vi "Meas_Fast_FID_Bkgnd.vi"(3 "Mode":T5, 5 "Traverse line In":T2 {"Carrier_2 Q (l/min)" format="%#.2f"; "Row Duration (mins)" format="%#.1f"; "Row No" min=0; "Trace Gas Concentration (%)" min=0.0 format="%#_4f"; "Carrier_1 Q (l/min)" format="%#.2f"; "Tunnel Speed" format="%#.2f"; "Start X" format="%#.2f"; "Start Y" format="%#.2f"; "Start Z" format="%#.2f"; "End X" format="%#.2f"; "End Y" format="%#.2f"; "End Z" format="%#.2f"; "Averaging time (min)" min=0.0 format="%#.2f"}) -> (0 "Error Message":string, 1 "Status":T1, 2 "Traverse line Out":T2 {"Carrier_2 Q (l/min)" format="%#.2f"; "Row Duration (mins)" format="%#.1f"; "Row No" min=0; "Trace Gas Concentration (%)" min=0.0 format="%#_4f"; "Carrier_1 Q (l/min)" format="%#.2f"; "Tunnel Speed" format="%#.2f"; "Start X" format="%#.2f"; "Start Y" format="%#.2f"; "Start Z" format="%#.2f"; "End X" format="%#.2f"; "End Y" format="%#.2f"; "End Z" format="%#.2f"; "Averaging time (min)" min=0.0 format="%#.2f"})   [LabVIEW 2015]
uses:
  Gen Trav/Traverse_cluster.ctl
  Gen Trav/Spacing.ctl
  Controls/Multi_run_mode.ctl
  Controls/User_Specific_mode.ctl
  Gen Trav/Multi_Run_Status.ctl
  File/Setup_Filetype.ctl
  Gen Trav/Trav_mode.ctl
  Controls/Home.ctl
  Controls/Setup.ctl
  Controls/Save_Data.ctl
  Globals/Trav_pos_global.vi
  Globals/Preference_global.vi
  Globals/Gas_management_global.vi
  Globals/Meas_global.vi
panel:
  out "Traverses":string[](array[string])
  out "Initial Trav Positions":sgl[][](array[numeric])
  out "First Bknd since calib":bool
  out "Initial Position":sgl[](array[numeric]) format="%#.2f"
  # "X           Y            Z"
  # "Start"
  # "End"
  # "X           Y            Z"
  # "Start"
  # "End"
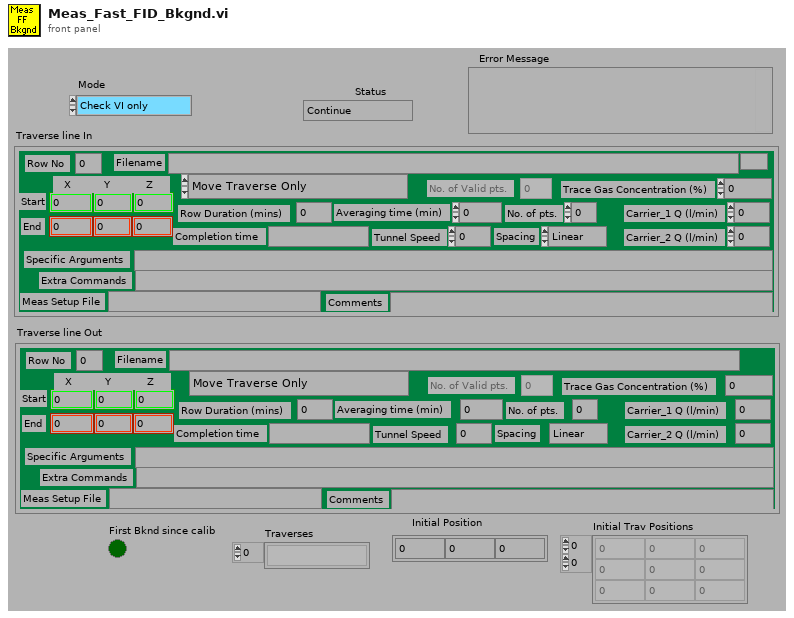
[diagram p1: front panel]
types:
  T1 = typedef "Multi_Run_Status.ctl" = enum16{"Continue", "Jump to Next Point", "Jump to Next Row", "Jump To Fall Back", "Terminate Run"}
  T2 = typedef "Traverse_cluster.ctl" = cluster{"Start X":sgl, "Start Y":sgl, "Start Z":sgl, "End X":sgl, "End Y":sgl, "End Z":sgl, "No. of pts.":i32, "Spacing":T3, "Filename":path, "Tunnel Speed":dbl, "Averaging time (min)":dbl, "Extra Commands":string, "Carrier_1 Q (l/min)":dbl, "Carrier_2 Q (l/min)":dbl, "Trace Gas Concentration (%)":dbl, "Specific Arguments":string, "Comments":string, "Row No":i32, "Row Type Selector":T4, "Completion time":string, "Row Duration (mins)":dbl, "No. of Valid pts.":i32, "Meas Setup File":string}
  T3 = typedef "Spacing.ctl" = enum16{"Linear", "Log", "Gauss", "Specified", "N/A"}
  T4 = typedef "Multi_run_mode.ctl" = enum16{"Move Traverse Only", "Set Tunnel Speed Only", "Set Source Only", "Set Measurement Conditions", "Single Measurement", "Vertical Profile", "Lateral Profile", "Longitudinal Profile", "Explore Volume", "Multi-Axis Profile", "Auto Calibrate", "Meas Fast FID Bkgnd", "Check Beam Power", "Scanning Valve Measurement", "Run VI Named:", "Set ADAM Ch", "Wait (minutes)", "Send Message", "Synchronize With:", "Fall Back to this Row", "Turn Off Row Repeating", "Blank Row", "Traverse 3D Volume"}
  T5 = typedef "User_Specific_mode.ctl" = enum16{"Check VI only", "Run VI"}
  T6 = typedef "Tunnel_Coordinates.ctl" = enum16{"Work in Tunnel Coordinates", "Work in Model Coordinates"}
  T7 = typedef "Setup_Filetype.ctl" = enum16{"Measurement Setups", "Calibration Setups", "General", "Results File Plotter Setups", "Speed Calib Tweaks"}
  T8 = typedef "Trav_mode.ctl" = enum16{"Move traverse", "Read traverse position", "Teach Position"}
  T9 = typedef "Home.ctl" = enum16{"Don't Home", "Home  +X", "Home  -X", "Home  +Y", "Home  -Y", "Home  +Z", "Home  -Z"}
  T10 = typedef "Save_Data.ctl" = enum16{"Save No Data", "Save Data"}
  T11 = typedef "Setup.ctl" = enum16{"Run Program", "Show Setup", "Save Current Setup", "Setup Front Panel"}
  T12 = typedef "Status_Cluster.ctl" = cluster{"Status":T1, "Error Type":string, "Error Description":string}
  T13 = typedef "Analysis_info_cluster.ctl" = cluster{"Colour":u32, "Inst type":T14, "Inst name":string, "Symbol":string, "Code name":string, "Extra Info":string, "Inst Array":T15, "Extra Titles":string[], "Extra Values":string[], "U":dbl, "u^2":dbl, "u^3":dbl, "u^4":dbl, "Skew_u":dbl, "Kurt_u":dbl, "Sd Error in Mean":dbl, "% u'/U":dbl, "X":dbl, "Y":dbl, "Z":dbl, "Timescale integral to 25%":dbl, "Sd Error in Variance":dbl, "Calib File":path, "Calib Constants":dbl[], "Output Position":bool, "Full Stats":bool, "Av Sampling Rate":dbl, "Av No of Samples":dbl, "Total Meas Time (s)":dbl, "ADAM Ch Name":string, "Max value":dbl, "Min value":dbl}
  T14 = typedef "Inst_type.ctl" = enum16{"Propeller anemometer", "Raw voltage", "Pressure Transducer", "Pitot-static tube", "Preston tube", "Hot wire", "Cross wire 1", "Cross wire 2", "Generic Linear", "Generic Polynomial", "Generic BackPoly", "Fast FID", "Thermocouple", "Cold wire", "Pulsed Wire", "LDA Vel", "LDA Tran time", "LDA Arr time", "Microphone"}
  T15 = typedef "Instrument_Array.ctl" = enum16{"PWA", "LDA", "Analogue"}
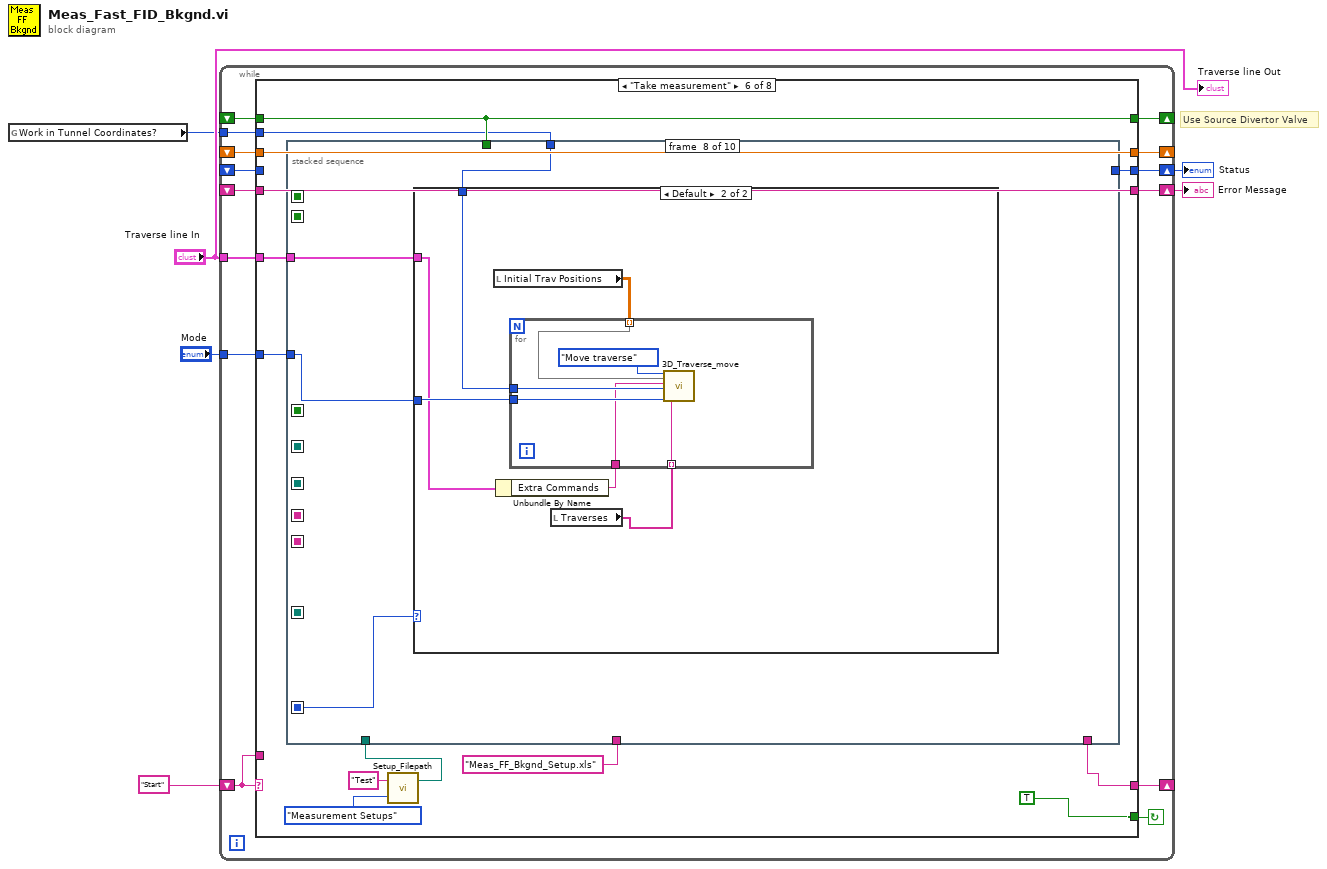
[diagram p0: block diagram]
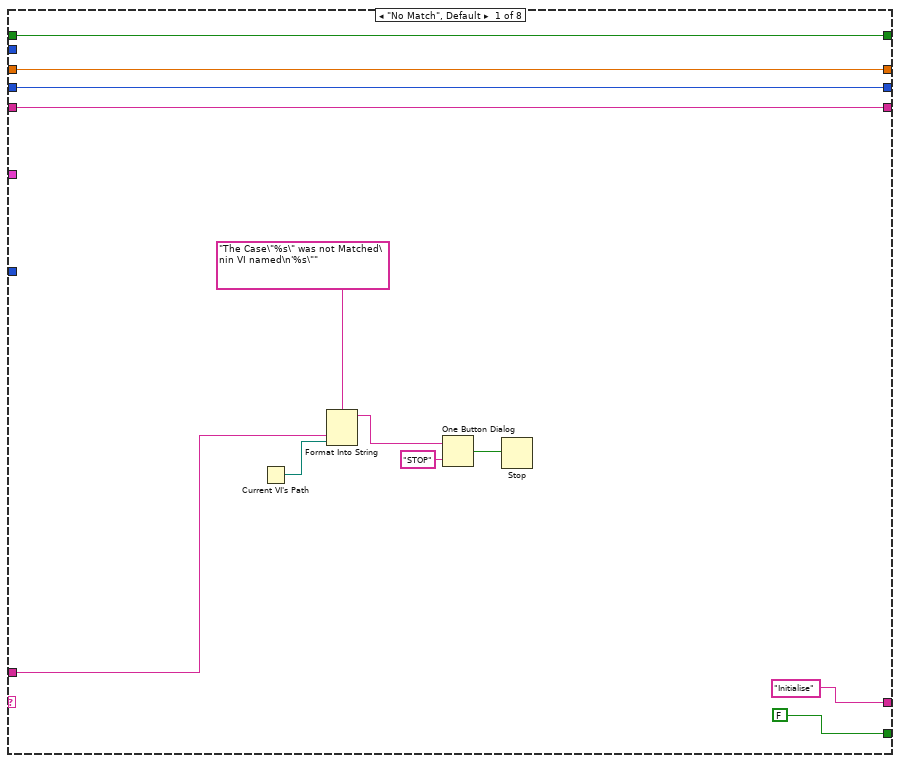
[diagram p2: hidden frame]
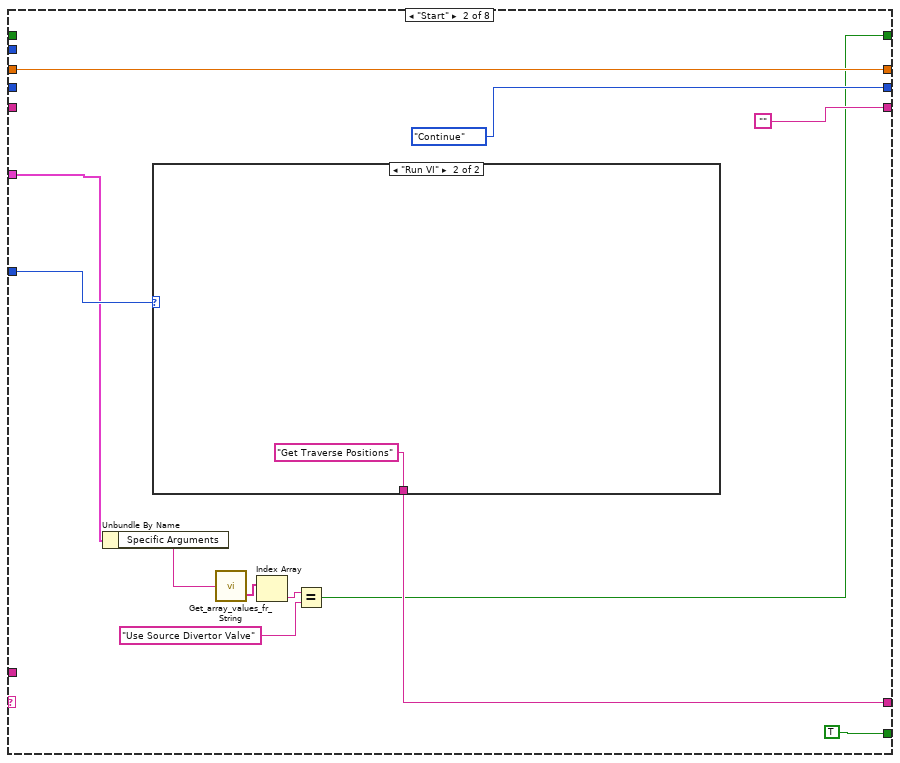
[diagram p3: hidden frame]
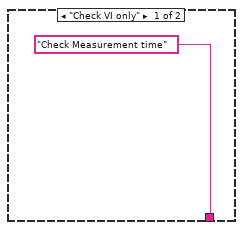
[diagram p4: hidden frame]
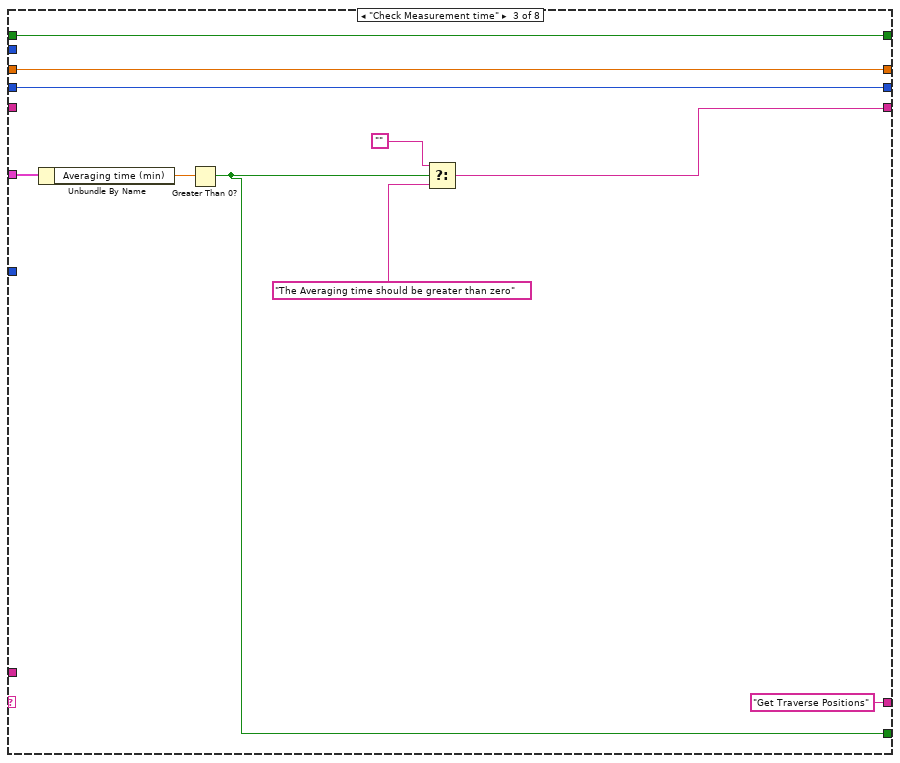
[diagram p5: hidden frame]
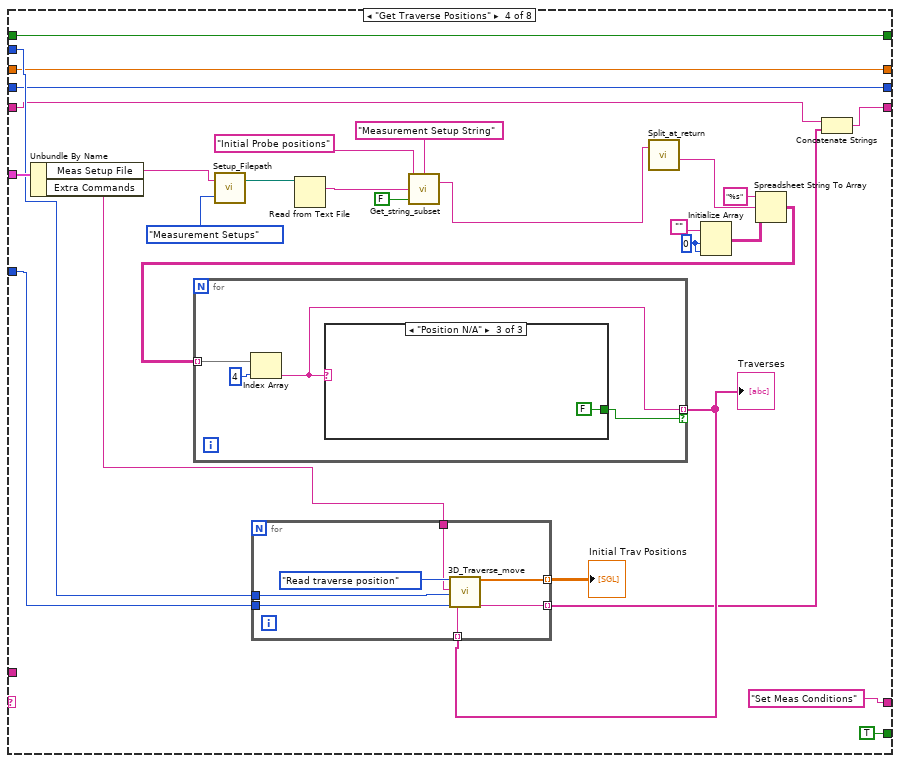
[diagram p6: hidden frame]
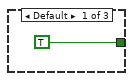
[diagram p7: hidden frame]
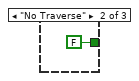
[diagram p8: hidden frame]
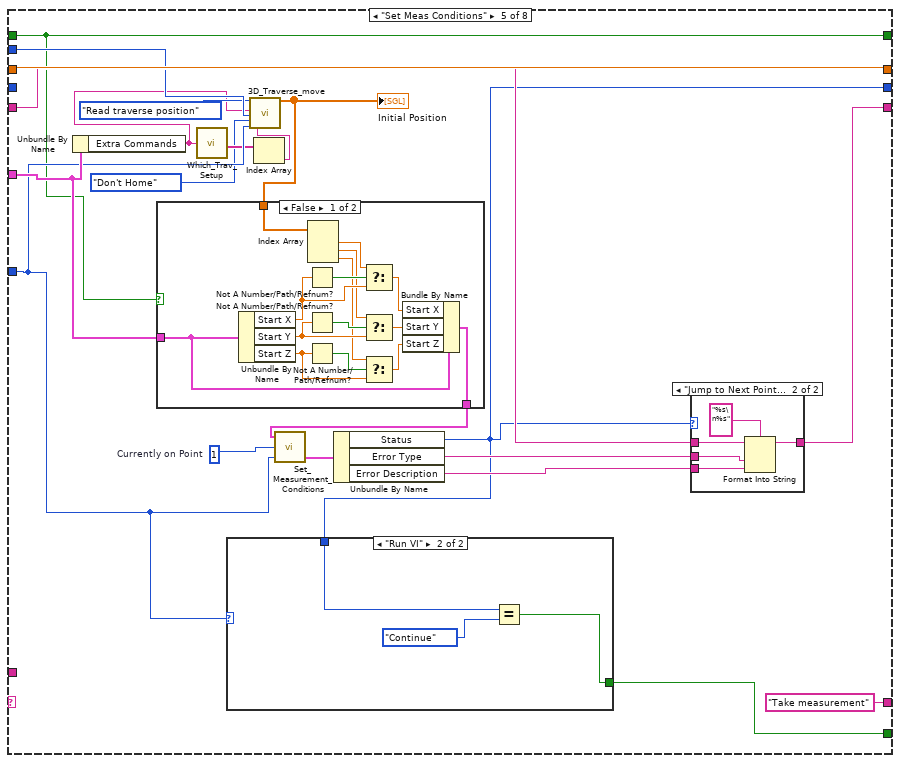
[diagram p9: hidden frame]
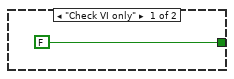
[diagram p12: hidden frame]
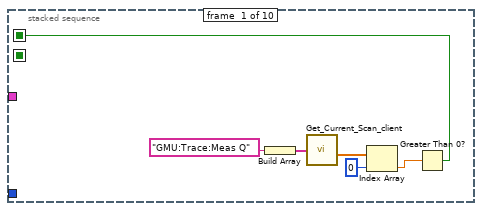
[diagram p13: hidden frame]
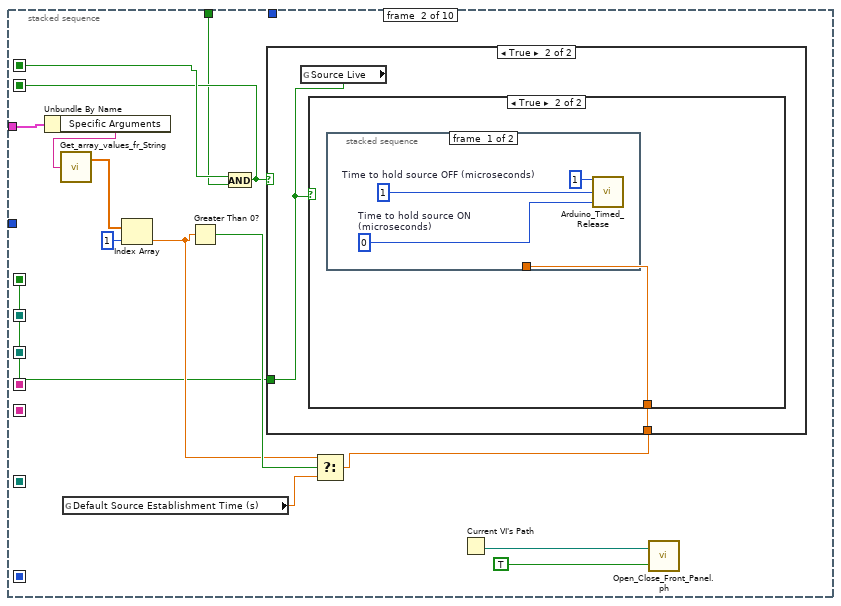
[diagram p14: hidden frame]
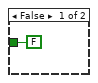
[diagram p15: hidden frame]
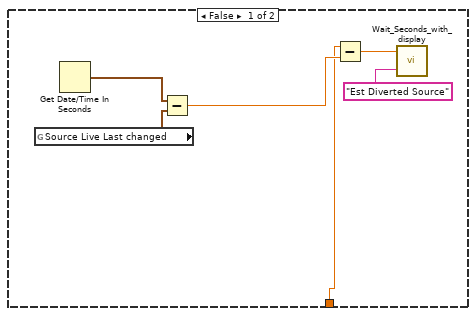
[diagram p16: hidden frame]
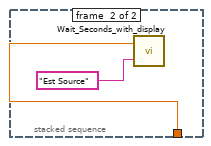
[diagram p17: hidden frame]
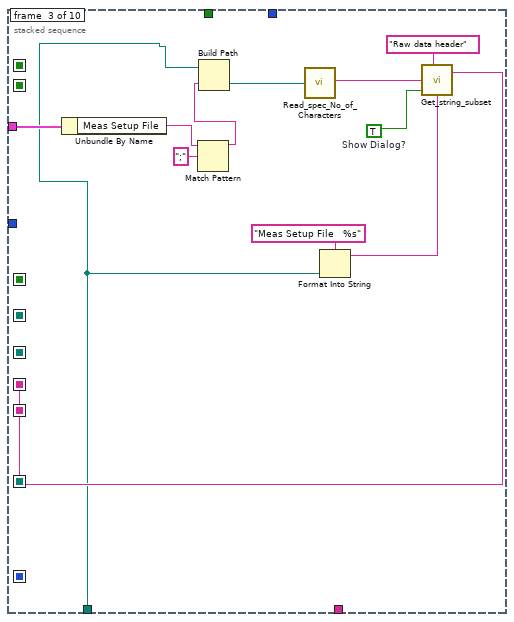
[diagram p18: hidden frame]
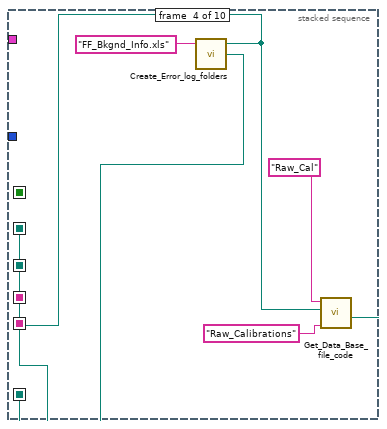
[diagram p19: hidden frame]
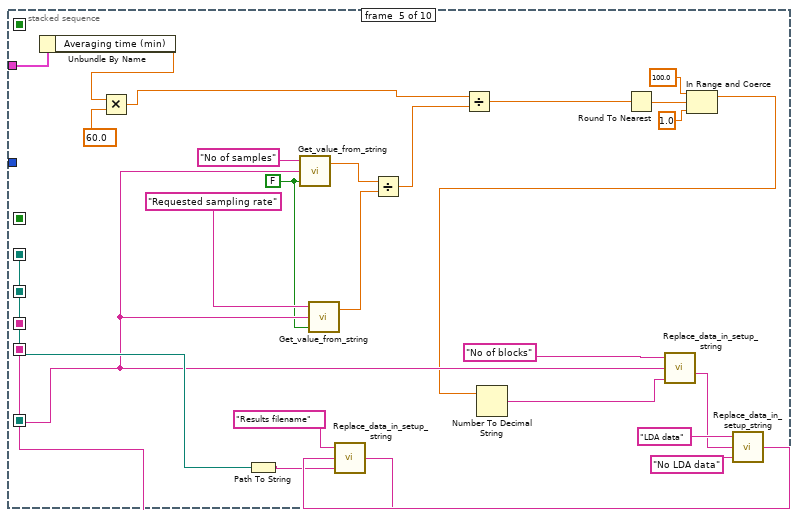
[diagram p20: hidden frame]
diagram:
  # "Use Source Divertor Valve"
  n1 = global read "Trav_pos_global.vi" "Work in Tunnel Coordinates?"() -> (w1:T6)
  n2 = while {
    shift-left: "Start" -> [w18]
    shift-right: [w19] -> _
    shift-right: [w14] -> _
    shift-left: _ -> [w17]
    tunnel: "Mode" -> [w16]
    tunnel: "Traverse line In" -> [w15]
    shift-right: [w13] -> w4
    shift-left: _ -> [w11]
    shift-right: [w12] -> w2
    shift-left: _ -> [w10]
    tunnel: w1 -> [w9]
    shift-right: [w7] -> _
    shift-left: _ -> [w8]
    stop <- w20 continue-if-true
    n3 = case shown="\"Take measurement\"" w18 {
      tunnel: [FALSE TRUE w50 TRUE w112 TRUE TRUE FALSE] -> w20
      tunnel: ["Initialise" w42 "Get Traverse Positions" "Set Meas Conditions" "Take measurement" ("t") w152 "Reset Measurement Program" "End"] -> w19
      tunnel: w18 -> [w27 _ _ _ _ _ _ _]
      tunnel: w17 -> [w24 w40 w48 w63 w117 w157 w393 _]
      tunnel: w16 -> [_ w43 _ w65 w108 w147 _ _]
      tunnel: w15 -> [_ w36 w56 w83 w109 w155 _ _]
      tunnel: [w24 w40 w48 w63 w117 w157 w393 w398] -> w14
      tunnel: [w23 Multi_Run_Status."Continue" ("Status") w49 w62 w110 w153 w392 w397] -> w13
      tunnel: [w22 "" w52 w59 w113 w156 w391 w400] -> w12
      tunnel: w11 -> [w23 _ w49 w62 _ _ w392 w397]
      tunnel: w10 -> [w22 _ _ w61 w114 w156 w391 w400]
      tunnel: w9 -> [_ _ _ w64 w107 w146 _ _]
      tunnel: w8 -> [w21 _ w47 w84 w99 w148 w388 w396]
      tunnel: [w21 w34 w47 w84 w99 w148 w388 w396] -> w7
      frame "No Match", Default {
        n4 = Current VI's Path() -> (path=w26:path)
        n5 = Format Into String(format string="The Case\"%s\" was not Matched\nin VI named\n'%s\"" ("Format String"), w27, w26) -> (resulting string=w30:string)  [unwired: 2 in, 1 out]
        n6 = One Button Dialog(message=w30, button name ("OK")="STOP") -> (true=w28:bool)
        n7 = Stop(stop? (T)=w28) -> ()
      }
      frame "Start" {
        n8 = Unbundle By Name(w36) -> ("Specific Arguments"=w35:string)
        n9 = case shown="\"Run VI\"" w43 {
          tunnel: ["Check Measurement time" "Get Traverse Positions"] -> w42
          frame "Check VI only" {
          }
          frame "Run VI" {
          }
        }
        n10 = call "Get_array_values_fr_String.vi"("String Value"=w35) -> ("String array"=w38:string[])  [unwired: 1 out]
        n11 = Index Array(array=w38) -> (element=w37:string)  [unwired: 1 in]
        n12 = Equal?(x=w37, y="Use Source Divertor Valve") -> (x = y?=w34:bool)
      }
      frame "Check Measurement time" {
        n13 = Unbundle By Name(w56) -> ("Averaging time (min)"=w55:dbl)
        n14 = Greater Than 0?(x=w55) -> (x > 0?=w50:bool)
        n15 = Select(t="", s=w50, f="The Averaging time should be greater than zero") -> (s? t:f=w52:string)
      }
      frame "Get Traverse Positions" {
        w77 = 0 ("Dimension Size")
        n16 = Unbundle By Name(w83) -> ("Meas Setup File"=w81:string, "Extra Commands"=w66:string)
        n17 = call "Setup_Filepath.vi"("Setup File Type"=Setup_Filetype."Measurement Setups", "Filename in"=w81) -> ("Directory"=w80:path)  [unwired: 1 out]
        n18 = Read from Text File(file (use dialog)=w80) -> (text=w70:string)  [unwired: 3 in, 3 out]
        n19 = call "Get_string_subset.vi"("String Name"="Measurement Setup String", "Show Dialog?"=FALSE, "String to split"=w70, "File Label"="Initial Probe positions") -> ("Output string"=w79:string)  [unwired: 1 out]
        n20 = call "Split_at_return.vi"("String"=w79) -> ("after substring"=w74:string)  [unwired: 1 in, 3 out]
        n21 = Initialize Array("", w77, w77) -> (w78:string[][])
        n22 = Spreadsheet String To Array(format string="%s", spreadsheet string=w74, array type (2D Dbl)=w78) -> (array=w69:string[][])  [unwired: 1 out]
        n23 = for {
          tunnel: w69 -> [w94] mode=indexing
          tunnel: [w93] -> w67 mode=indexing if=w92
          n24 = Index Array(array=w94, index=4) -> (element=w93:string)
          n25 = case shown="\"Position N/A\"" w93 {
            tunnel: [TRUE FALSE FALSE] -> w92
            frame Default {
            }
            frame "No Traverse" {
            }
            frame "Position N/A" {
            }
          }
        }
        "Traverses" <- w67
        n26 = for {
          tunnel: w67 -> [w90] mode=indexing
          tunnel: w64 -> [w89]
          tunnel: w66 -> [w88]
          tunnel: w65 -> [w87]
          tunnel: [w86] -> w68 mode=indexing
          tunnel: [w85] -> w60 mode=indexing
          n27 = call "3D_Traverse_move.vi"("Mode"=Trav_mode."Read traverse position", "Extra command String"=w88, "Work in Tunnel Coordinates"=w89, "Simulate/Run"=w87, "Traverse name"=w90) -> ("Trav Position achieved"=w86:sgl[], "Error String"=w85:string)  [unwired: 12 in, 1 out]
        }
        "Initial Trav Positions" <- w68
        n28 = Concatenate Strings(w61, w60) -> (w59:string)
      }
      frame "Set Meas Conditions" {
        w119 = 1  # Currently on Point
        n29 = Unbundle By Name(w109) -> ("Extra Commands"=w100:string)
        n30 = call "Which_Trav_Setup.vi"("Extra Command String"=w100) -> ("Traverse Setups"=w103:string[])
        n31 = Index Array(array=w103) -> (element=w102:string)  [unwired: 1 in]
        n32 = call "3D_Traverse_move.vi"("Mode"=Trav_mode."Read traverse position", "Extra command String"=w100, "Work in Tunnel Coordinates"=w107, "Home"=Home."Don't Home", "Simulate/Run"=w108, "Traverse name"=w102) -> ("Trav Position achieved"=w104:sgl[])  [unwired: 11 in, 2 out]
        "Initial Position" <- w104
        n33 = case shown="False" w99 {
          tunnel: w109 -> [w134 w135]
          tunnel: [w133 w135] -> w106
          tunnel: w104 -> [w132 _]
          frame False {
            n34 = Unbundle By Name(w134) -> ("Start X"=w128:sgl, "Start Y"=w124:sgl, "Start Z"=w123:sgl)
            n35 = Not A Number/Path/Refnum?(number/path/refnum=w128) -> (NaN/Path/Refnum?=w131:bool)
            n36 = Not A Number/Path/Refnum?(number/path/refnum=w124) -> (NaN/Path/Refnum?=w127:bool)
            n37 = Not A Number/Path/Refnum?(number/path/refnum=w123) -> (NaN/Path/Refnum?=w126:bool)
            n38 = Index Array(array=w132) -> (element #1=w129:sgl, element #2=w122:sgl, element #3=w121:sgl)  [unwired: 3 in]
            n39 = Select(t=w129, s=w131, f=w128) -> (s? t:f=w130:sgl)
            n40 = Select(t=w122, s=w127, f=w124) -> (s? t:f=w125:sgl)
            n41 = Select(t=w121, s=w126, f=w123) -> (s? t:f=w120:sgl)
            n42 = Bundle By Name(cluster=w134, "Start X"=w130, "Start Y"=w125, "Start Z"=w120) -> (w133:T2)
          }
          frame True {
          }
        }
        n43 = call "Set_Measurement_Conditions.vi"("Simulate/Run"=w108, "Currently on Point"=w119, "Traverse line"=w106) -> ("Status Cluster"=w118:T12)  [unwired: 2 out]
        n44 = Unbundle By Name(w118) -> ("Status"=w110:T1, "Error Type"=w116:string, "Error Description"=w115:string)
        n45 = case shown="\"Run VI\"" w108 {
          tunnel: [FALSE w144] -> w112
          tunnel: w110 -> [_ w145]
          frame "Check VI only" {
          }
          frame "Run VI" {
            n46 = Equal?(x=w145, y=Multi_Run_Status."Continue" ("Status")) -> (x = y?=w144:bool)
          }
        }
        n47 = case shown="\"Jump to Next Point\", Default" w110 {
          tunnel: w116 -> [_ w141]
          tunnel: w115 -> [_ w140]
          tunnel: w114 -> [w136 w139]
          tunnel: [w136 w138] -> w113
          frame "Continue" {
          }
          frame "Jump to Next Point", Default {
            n48 = Format Into String(format string="%s\n%s", initial string=w139, w141, w140) -> (resulting string=w138:string)  [unwired: 1 in, 1 out]
          }
        }
      }
      frame "Take measurement" {
        n49 = call "Setup_Filepath.vi"("Setup File Type"=Setup_Filetype."Measurement Setups", "Filename in"="Test") -> ("Directory"=w149:path)  [unwired: 1 out]
        n50 = stacked-sequence {
          seq-local: [_ _ w203 _ _ _ _ _ _ _] -> [_ _ _ _ w219 _ _ _ _ _]
          seq-local: [_ _ _ _ w228 _ _ _ _ _] -> [_ _ _ _ _ w240 _ _ _ _]
          seq-local: [_ _ _ w208 _ _ _ _ _ _] -> [_ _ _ _ _ _ w259 _ _ _]
          seq-local: [_ _ _ w210 _ _ _ _ _ _] -> [_ _ _ _ w227 _ _ _ w372 _]
          seq-local: [_ w167 _ _ _ _ _ _ _ _] -> [_ _ _ _ _ _ _ _ _ _]
          seq-local: [_ _ _ w207 _ _ _ _ _ _] -> [_ _ _ _ _ _ _ _ w371 _]
          seq-local: [w159 _ _ _ _ _ _ _ _ _] -> [_ w168 _ _ _ _ _ _ _ _]
          seq-local: [_ w165 _ _ _ _ _ _ _ _] -> [_ _ _ _ _ _ _ _ w370 _]
          seq-local: [_ _ _ _ _ _ w249 _ _ _] -> [_ _ _ _ _ _ _ w357 _ _]
          tunnel: "Meas_FF_Bkgnd_Setup.xls" -> [_ _ _ _ _ w242 w260 _ _ _]
          tunnel: w155 -> [_ w176 w200 _ w223 _ w252 w356 _ w378]
          tunnel: [_ _ _ _ _ _ w258 _ _ _] -> w153
          tunnel: [_ _ _ _ _ _ w256 _ _ _] -> w152
          tunnel: w149 -> [_ _ w195 _ _ w238 _ _ _ _]
          tunnel: w148 -> [_ w166 _ _ _ _ _ _ _ _]
          tunnel: w147 -> [_ _ _ _ _ _ w250 w355 _ w377]
          tunnel: w146 -> [_ _ _ _ _ _ w251 w354 _ _]
          frame #0 {
            n51 = Build Array("GMU:Trace:Meas Q") -> (w163:string[])
            n52 = call "Get_Current_Scan_client.vi"("ADAM Ch Names"=w163) -> ("Numerical Values"=w161:dbl[])  [unwired: 3 out]
            n53 = Index Array(array=w161, index=0) -> (element=w160:dbl)
            n54 = Greater Than 0?(x=w160) -> (x > 0?=w159:bool)
          }
          frame #1 {
            n55 = Unbundle By Name(w176) -> ("Specific Arguments"=w175:string)
            n56 = call "Get_array_values_fr_String.vi"("String Value"=w175) -> ("Numeric Array"=w173:dbl[])  [unwired: 1 out]
            n57 = global read "Preference_global.vi" "Default Source Establishment Time (s)"() -> (w170:dbl)
            n58 = Index Array(array=w173, index=1) -> (element=w171:dbl)
            n59 = Greater Than 0?(x=w171) -> (x > 0?=w172:bool)
            n60 = And(x=w168, y=w166) -> (x .and. y?=w167:bool)
            n61 = Select(t=w171, s=w172, f=w170) -> (s? t:f=w169:dbl)
            n62 = case shown="True" w167 {
              tunnel: w169 -> [_ w181]
              tunnel: [FALSE w180] -> w165
              frame False {
              }
              frame True {
                n63 = global read "Gas_management_global.vi" "Source Live"() -> (w180:bool)
                n64 = case shown="True" w180 {
                  tunnel: w181 -> [w182 w188]
                  frame False {
                    n65 = global read "Gas_management_global.vi" "Source Live Last changed"() -> (w184:timestamp)
                    n66 = Get Date/Time In Seconds() -> (seconds since 1Jan1904=w183:timestamp)
                    n67 = Subtract(x=w183, y=w184) -> (x-y=w185:dbl)
                    n68 = Subtract(x=w182, y=w185) -> (x-y=w187:dbl)
                    n69 = call "Wait_Seconds_with_display.vi"("Message"="Est Diverted Source", "Seconds to wait"=w187) -> ()  [unwired: 2 out]
                  }
                  frame True {
                    n70 = stacked-sequence {
                      tunnel: w188 -> [_ w192]
                      frame #0 {
                        w189 = u32 1  # Time to hold source OFF (microseconds)
                        w190 = u32 0  # Time to hold source ON (microseconds)
                        n71 = call "Arduino_Timed_Release.vi"("Time to hold source ON (microseconds)"=w190, "Time to hold source OFF (microseconds)"=w189, "Number of cycles"=u16 1) -> ()  [unwired: 2 out]
                      }
                      frame #1 {
                        n72 = call "Wait_Seconds_with_display.vi"("Message"="Est Source", "Seconds to wait"=w192) -> ()  [unwired: 2 out]
                      }
                    }
                  }
                }
              }
            }
            n73 = Current VI's Path() -> (path=w177:path)
            n74 = call "Open_Close_Front_Panel.ph.vi"("Front Panel Window:Open"=TRUE, "VI path"=w177) -> ()  [unwired: 2 out]
          }
          frame #2 {
            w201 = TRUE  # Show Dialog?
            n75 = Unbundle By Name(w200) -> ("Meas Setup File"=w198:string)
            n76 = Match Pattern(string=w198, regular expression=";") -> (before substring=w197:string)  [unwired: 4 out]
            n77 = Build Path(base path=w195, name or relative path=w197) -> (appended path=w202:path)
            n78 = call "Read_spec_No_of_Characters.vi"("Filename"=w202) -> ("character string"=w204:string)  [unwired: 1 out]
            n79 = Format Into String(format string="Meas Setup File   %s", w195) -> (resulting string=w194:string)  [unwired: 2 in, 1 out]
            n80 = call "Get_string_subset.vi"("String Name"=w194, "Show Dialog?"=w201, "String to split"=w204, "File Label"="Raw data header") -> ("Output string"=w203:string)  [unwired: 1 out]
          }
          frame #3 {
            n81 = call "Create_Error_log_folders.vi"("Log Filename"="FF_Bkgnd_Info.xls") -> ("Server copy Location"=w207:path, "Local Log File"=w210:path)  [unwired: 2 in, 1 out]
            n82 = call "Get_Data_Base_file_code.vi"("Data Type"="Raw_Calibrations", "Results Filename"=w210, "Short_Name"="Raw_Cal") -> ("Raw Data File Name"=w208:path)  [unwired: 1 in, 3 out]
          }
          frame #4 {
            w216 = FALSE ("Show Dialog?")
            n83 = Unbundle By Name(w223) -> ("Averaging time (min)"=w222:dbl)
            n84 = Multiply(x=w222, y=60.0) -> (x*y=w224:dbl)
            n85 = Path To String(path=w227) -> (string=w226:string)
            n86 = call "Get_value_from_string.vi"("Show Dialog?"=w216, "Input string"=w219, "Variable name"="No of samples") -> ("Value"=w217:dbl)  [unwired: 1 out]
            n87 = call "Get_value_from_string.vi"("Show Dialog?"=w216, "Input string"=w219, "Variable name"="Requested sampling rate") -> ("Value"=w218:dbl)  [unwired: 1 out]
            n88 = Divide(x=w217, y=w218) -> (x/y=w237:dbl)
            n89 = Divide(x=w224, y=w237) -> (x/y=w236:dbl)
            n90 = Round To Nearest(number=w236) -> (nearest integer value=w215:dbl)
            n91 = In Range and Coerce(upper limit=100.0, x=w215, lower limit=1.0) -> (coerced(x)=w212:dbl)  [unwired: 1 out]
            n92 = Number To Decimal String(number=w212) -> (decimal integer string=w234:string)  [unwired: 1 out]
            n93 = call "Replace_data_in_setup_string.vi"("New data string"=w234, "Input string"=w219, "Variable name"="No of blocks") -> ("Appended string"=w231:string)
            n94 = call "Replace_data_in_setup_string.vi"("New data string"="No LDA data", "Input string"=w231, "Variable name"="LDA data" ("Label for characters")) -> ("Appended string"=w229:string)
            n95 = call "Replace_data_in_setup_string.vi"("New data string"=w226, "Input string"=w229, "Variable name"="Results filename") -> ("Appended string"=w228:string)
          }
          frame #5 {
            w246 = FALSE  # advisory dialog? (display:T)
            w247 = FALSE  # append to file? (new file:F)
            n96 = call "Remove_Plug_Ins_etc.vi"("Input String"=w240) -> ("Output string"=w239:string)
            n97 = call "Add_label_to_string.vi"("String to write"=w239, "File Label"="Raw data header") -> ("Output string"=w243:string)
            n98 = Build Path(base path=w238, name or relative path=w242) -> (appended path=w241:path)
            n99 = call "Add_length_to_string.vi"("String in"=w243) -> ("String out"=w245:string)
            n100 = call "Write_Characters_To_File.vi"("file path (dialog if empty)"=w241, "advisory dialog? (display:T)"=w246, "character string"=w245, "append to file? (new file:F)"=w247) -> ()  [unwired: 1 in, 4 out]
          }
          frame #6 {
            n101 = for {
              N: 4 -> [_]
              tunnel: w260 -> [w270]
              tunnel: w259 -> [w269]
              tunnel: [w268] -> w258
              tunnel: [w267] -> w257
              tunnel: w252 -> [w265]
              tunnel: w251 -> [w264]
              tunnel: w250 -> [w263]
              tunnel: [w262] -> w249
              tunnel: [w261] -> w248
              i -> [w262]
              stop <- w266 continue-if-true
              n102 = stacked-sequence {
                seq-local: [w273 _ _ _ _] -> [_ _ w308 _ _]
                seq-local: [_ _ w307 _ _] -> [_ _ _ w313 w331]
                seq-local: [_ w284 _ _ _] -> [_ _ w306 _ _]
                tunnel: w270 -> [w279 _ _ _ _]
                tunnel: w269 -> [w277 _ _ _ _]
                tunnel: [w275 _ _ _ _] -> w268
                tunnel: [w273 _ _ _ _] -> w267
                tunnel: [_ _ w307 _ _] -> w266
                tunnel: w265 -> [w271 _ _ w312 w330]
                tunnel: w264 -> [_ _ _ w311 w329]
                tunnel: w263 -> [_ _ _ w310 w328]
                tunnel: w262 -> [_ _ _ w309 w327]
                tunnel: [_ w282 _ _ _] -> w261
                frame #0 {
                  w281 = TRUE  # Remote control
                  n103 = Unbundle By Name(w271) -> ("Extra Commands"=w272:string)
                  n104 = call "Code_to_run.vi"("Extra command String"=w272, "Raw data option"=enum16{"Save raw data", "Raw data not saved"}."Save raw data", "setup"=Setup."Run Program", "Remote control"=w281, "File"=Save_Data."Save Data", "Raw data file"=w277, "Setup filename"=w279) -> ("Status"=w275:T1)  [unwired: 5 in, 3 out]
                  n105 = Equal?(x=w275, y=Multi_Run_Status."Continue" ("Status")) -> (x = y?=w273:bool)
                }
                frame #1 {
                  n106 = global read "Meas_global.vi" "Analysis Info cluster"() -> (w286:T13[])
                  n107 = for {
                    tunnel: w286 -> [w289] mode=indexing
                    tunnel: [w288] -> w285 mode=indexing
                    tunnel: [w287] -> w283 mode=indexing
                    n108 = Unbundle By Name(w289) -> ("Inst type"=w290:T14)
                    n109 = case shown="\"Fast FID\"" w290 {
                      tunnel: w289 -> [_ w305]
                      tunnel: [FALSE w294] -> w288
                      tunnel: [FALSE w293] -> w287
                      frame Default {
                      }
                      frame "Fast FID" {
                        n110 = Unbundle By Name(w305) -> ("u^2"=w300:dbl, "Calib Constants"=w301:dbl[])
                        n111 = Index Array(array=w301, index=3 ("Index")) -> (element=w303:dbl)
                        n112 = Index Array(array=w301, index=4) -> (element=w297:dbl)
                        n113 = Equal To 0?(x=w303) -> (x = 0?=w293:bool)
                        n114 = Multiply(x=w297, y=1.4) -> (x*y=w295:dbl)
                        n115 = Select(t=1.5 ("y"), s=w293, f=w295) -> (s? t:f=w298:dbl)
                        n116 = Greater?(x=w300, y=w298) -> (0:w294:bool)
                      }
                    }
                  }
                  n117 = Or Array Elements(Boolean array=w285) -> (logical OR=w284:bool)
                  n118 = Or Array Elements(Boolean array=w283) -> (logical OR=w282:bool)
                }
                frame #2 {
                  n119 = Compound Arithmetic op=AND(w306, w308) -> (w307:bool)
                }
                frame #3 {
                  n120 = case shown="True" w313 {
                    tunnel: w312 -> [_ w323]
                    tunnel: w311 -> [_ _]
                    tunnel: w310 -> [_ w321]
                    tunnel: w309 -> [_ w316]
                    frame False {
                    }
                    frame True {
                      w326 = 1  # Currently on Point
                      n121 = Increment(x=w316) -> (x+1=w315:i32)
                      n122 = local read "Initial Position"() -> (w318:sgl[])
                      n123 = Multiply(x=w315, y=sgl 100.0) -> (x*y=w314:sgl)
                      n124 = Index Array(array=w318) -> (element #1=w325:sgl, element #2=w324:sgl, element #3=w320:sgl)  [unwired: 3 in]
                      n125 = Add(x=w320, y=w314) -> (x+y=w319:sgl)
                      n126 = Bundle By Name(cluster=w323, "Start X"=w325, "Start Y"=w324, "Start Z"=w319) -> (w322:T2)
                      n127 = call "Set_Measurement_Conditions.vi"("Simulate/Run"=w321, "Currently on Point"=w326, "Traverse line"=w322) -> ()  [unwired: 3 out]
                    }
                  }
                }
                frame #4 {
                  n128 = case shown="True" w331 {
                    tunnel: w330 -> [_ w333]
                    tunnel: w329 -> [_ w336]
                    tunnel: w328 -> [_ w335]
                    tunnel: w327 -> [_ w339]
                    frame False {
                    }
                    frame True {
                      n129 = local read "Initial Trav Positions"() -> (w337:sgl[][])
                      n130 = Increment(x=w339) -> (x+1=w338:i32)
                      n131 = Unbundle By Name(w333) -> ("Extra Commands"=w332:string)
                      n132 = local read "Traverses"() -> (w334:string[])
                      n133 = for {
                        tunnel: w338 -> [w349]
                        tunnel: w337 -> [w346] mode=indexing
                        tunnel: w336 -> [w344]
                        tunnel: w335 -> [w343]
                        tunnel: w334 -> [w342] mode=indexing
                        tunnel: w332 -> [w340]
                        n134 = Multiply(x=w349, y=sgl 100.0) -> (x*y=w347:sgl)
                        n135 = in-place {
                          in-place-border: w347 -> [w352]
                          n136 = in-place-array #1(w346, 2) -> (w353:sgl)
                          n137 = Add(x=w353, y=w352) -> (x+y=w351:sgl)
                          n138 = in-place-array #1(w351) -> (w345:sgl[])  [unwired: 1 out]
                        }
                        n139 = call "3D_Traverse_move.vi"("Mode"=Trav_mode."Move traverse", "Position"=w345, "Extra command String"=w340, "Work in Tunnel Coordinates"=w344, "Simulate/Run"=w343, "Traverse name"=w342) -> ()  [unwired: 11 in, 3 out]
                      }
                    }
                  }
                }
              }
            }
            "First Bknd since calib" <- w248
            n140 = Select(t="Update calib files", s=w257, f="Reset Measurement Program") -> (s? t:f=w256:string)
          }
          frame #7 {
            n141 = case shown="Default" w357 {
              tunnel: w356 -> [_ w359]
              tunnel: w355 -> [_ w362]
              tunnel: w354 -> [_ w361]
              frame 0 {
              }
              frame Default {
                n142 = local read "Initial Trav Positions"() -> (w360:sgl[][])
                n143 = Unbundle By Name(w359) -> ("Extra Commands"=w358:string)
                n144 = local read "Traverses"() -> (w363:string[])
                n145 = for {
                  tunnel: w363 -> [w369] mode=indexing
                  tunnel: w362 -> [w368]
                  tunnel: w361 -> [w367]
                  tunnel: w360 -> [w365] mode=indexing
                  tunnel: w358 -> [w364]
                  n146 = call "3D_Traverse_move.vi"("Mode"=Trav_mode."Move traverse", "Position"=w365, "Extra command String"=w364, "Work in Tunnel Coordinates"=w367, "Simulate/Run"=w368, "Traverse name"=w369) -> ()  [unwired: 11 in, 3 out]
                }
              }
            }
          }
          frame #8 {
            n147 = call "Updated_File_Copy.vi"("Target Path"=w371, "Source Path"=w372) -> ()  [unwired: 2 out]
            n148 = case shown="True" w370 {
              frame False {
              }
              frame True {
                w373 = u32 0  # Time to hold source OFF (microseconds)
                w374 = u32 1  # Time to hold source ON (microseconds)
                n149 = call "Arduino_Timed_Release.vi"("Time to hold source ON (microseconds)"=w374, "Time to hold source OFF (microseconds)"=w373, "Number of cycles"=u16 1) -> ()  [unwired: 2 out]
              }
            }
          }
          frame #9 {
            n150 = case shown="True" FALSE {
              tunnel: w378 -> [_ w381]
              tunnel: w377 -> [_ w379]
              frame False {
              }
              frame True {
                w386 = 1  # Currently on Point
                n151 = local read "Initial Position"() -> (w385:sgl[])
                n152 = Index Array(array=w385) -> (element #1=w384:sgl, element #2=w383:sgl, element #3=w382:sgl)  [unwired: 3 in]
                n153 = Bundle By Name(cluster=w381, "Start X"=w384, "Start Y"=w383, "Start Z"=w382) -> (w380:T2)
                n154 = call "Set_Measurement_Conditions.vi"("Simulate/Run"=w379, "Currently on Point"=w386, "Traverse line"=w380) -> ()  [unwired: 3 out]
              }
            }
          }
        }
      }
      frame "Update calib files" {
        w389 = dbl[] [] ("C (ppm)")
        w390 = TRUE  # Specific Bkgnd Meas?
        n155 = local read "First Bknd since calib"() -> (w387:bool)
        n156 = call "Update_FFID_Bkgnd_info.vi"("First Bknd since calib"=w387, "c^2 (ppm^2)"=w389, "Specific Bkgnd Meas?"=w390, "C (ppm)"=w389) -> ()  [unwired: 1 in]
      }
      frame "Reset Measurement Program" {
        n157 = Get Date/Time In Seconds() -> (seconds since 1Jan1904=w399:timestamp)
        n158 = To Double Precision Float(number=w399) -> (double precision float=w398:dbl)
      }
    }
  }
  "Error Message" <- w2
  "Status" <- w4
  "Traverse line Out" <- "Traverse line In"
